vi "PositionLabelsInPlace.vi"(8 "error in (no error)":errorcluster, 11 "XYGraph in":refnum<vi>) -> (0 "error out":errorcluster)   [LabVIEW 2022 SP3, in "PentaPanesLibrary.lvlib" / "PentaPanes.lvclass"]
uses:
  PentaPanes.lvclass
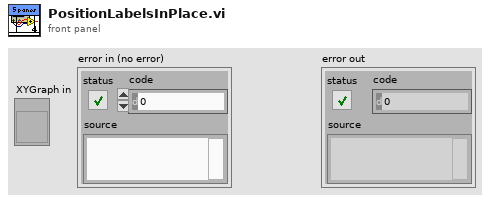
[diagram p1: front panel]
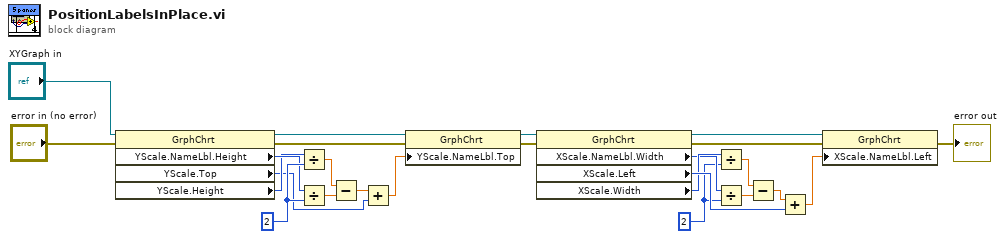
[diagram p0: block diagram]
diagram:
  w11 = u32 2 ("y")
  w16 = u32 2 ("y")
  n1 = property class="GrphChrt"(reference="XYGraph in", error in="error in (no error)") -> (reference out=w6:refnum<vi>, error out=w3:errorcluster, "YScale.NameLbl.Height"=w10:u32, "YScale.Top"=w8:i32, "YScale.Height"=w9:u32)
  n2 = Divide(x=w9, y=w11) -> (x/y=w12:dbl)
  n3 = Divide(x=w10, y=w11) -> (x/y=w13:dbl)
  n4 = Subtract(x=w12, y=w13) -> (x-y=w14:dbl)
  n5 = Add(x=w14, y=w8) -> (x+y=w15:dbl)
  n6 = property class="GrphChrt"(reference=w6, error in=w3, "YScale.NameLbl.Top"=w15) -> (reference out=w5:refnum<vi>, error out=w4:errorcluster)
  n7 = property class="GrphChrt"(reference=w5, error in=w4) -> (reference out=w20:refnum<vi>, error out=w21:errorcluster, "XScale.NameLbl.Width"=w19:u32, "XScale.Left"=w25:i32, "XScale.Width"=w22:u32)
  n8 = Divide(x=w22, y=w16) -> (x/y=w17:dbl)
  n9 = Divide(x=w19, y=w16) -> (x/y=w18:dbl)
  n10 = Subtract(x=w17, y=w18) -> (x-y=w23:dbl)
  n11 = Add(x=w23, y=w25) -> (x+y=w24:dbl)
  n12 = property class="GrphChrt"(reference=w20, error in=w21, "XScale.NameLbl.Left"=w24) -> (error out=→"error out":errorcluster)  [unwired: 1 out]
